vi "Auto Match.vi"() -> ()   [LabVIEW 2014]
doc: "This VI is used to demonstrate passing data out of a while loop through a tunnel. This VI generates random numbers until the generated number matches a specified value. The loop count terminal keeps track of the number of iterations before a match occurs."
panel:
  out "Number of Iterations":i32
  out "Current Number":u32 format="%#.0f"
  in  "Number to Match":u32=50 max=1000 step=1
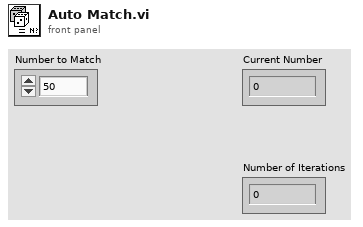
[diagram p1: front panel]
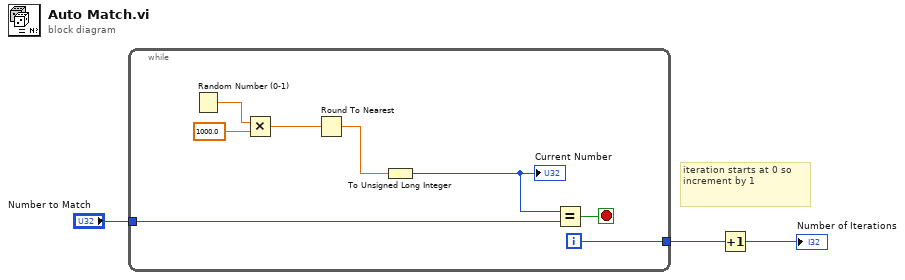
[diagram p0: block diagram]
diagram:
  # "iteration starts at 0 so increment by 1"
  n1 = while {
    tunnel: [w7] -> w3
    tunnel: "Number to Match" -> [w6]
    i -> [w7]
    stop <- w8 stop-if-true
    n2 = Random Number (0-1)() -> (number: 0 to 1=w9:dbl)
    n3 = Multiply(x=w9, y=1000.0) -> (x*y=w11:dbl)
    n4 = Round To Nearest(number=w11) -> (nearest integer value=w5:dbl)
    n5 = To Unsigned Long Integer(number=w5) -> (unsigned 32bit integer=w4:u32)
    "Current Number" <- w4
    n6 = Equal?(x=w4, y=w6) -> (x = y?=w8:bool)
  }
  n7 = Increment(x=w3) -> (x+1=→"Number of Iterations":i32)
